vi "Write Identity Toolkit URL.vi"(8 "error in (no error)":errorcluster, 10 "Identity Toolkit URL":string, 11 "firebase in":refnum<class "firebase.lvclass">) -> (0 "error out":errorcluster, 3 "firebase out":refnum<class "firebase.lvclass">)   [LabVIEW 2019, in "firebase.lvclass"]
uses:
  firebase.lvclass
  firebase.lvclass/firebase.ctl
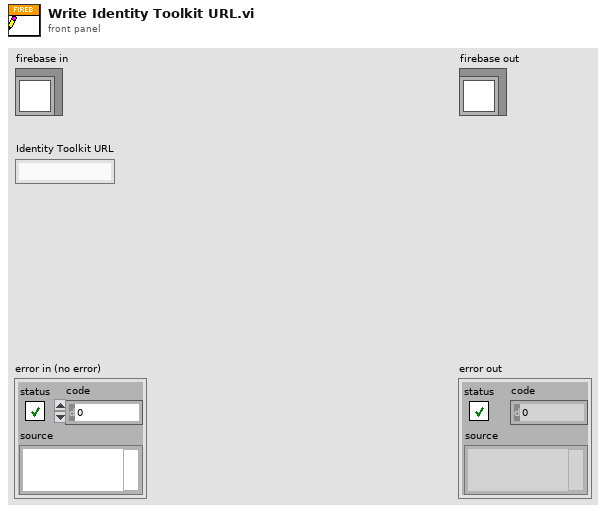
[diagram p1: front panel]
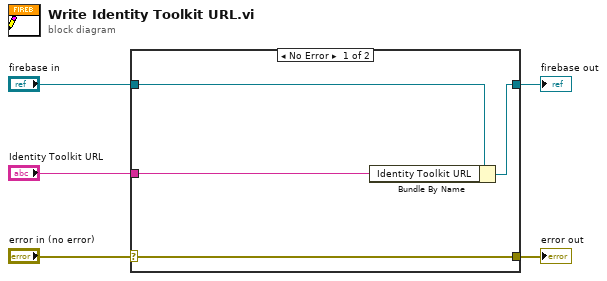
[diagram p0: block diagram]
diagram:
  n1 = case shown="No Error" "error in (no error)" {
    selector: "error in (no error)" -> [w9 w10]
    tunnel: [w9 w10] -> w4
    tunnel: [w7 w11] -> w2
    tunnel: "firebase in" -> [w8 w11]
    tunnel: "Identity Toolkit URL" -> [w6 _]
    frame No Error {
      n2 = Bundle By Name(cluster=w8, "Identity Toolkit URL"=w6) -> (w7:refnum<class "firebase.lvclass">)
    }
    frame Error {
    }
  }
  "error out" <- w4
  "firebase out" <- w2
